vi "AudioTest.Load All Plot Limit Definition Files.vi"(8 "error in (no error)":errorcluster, 11 "Config Folder":path=path "C:/MTE/Audio Test/Config") -> (0 "error out":errorcluster, 3 "LimitPlots":T1[](array[typedef]))   [LabVIEW 2018]
uses:
  TypeDefs/AudioTest.Result Plot Data.ctl
  <vilib>/KATE/Files/File Utils.lvlib
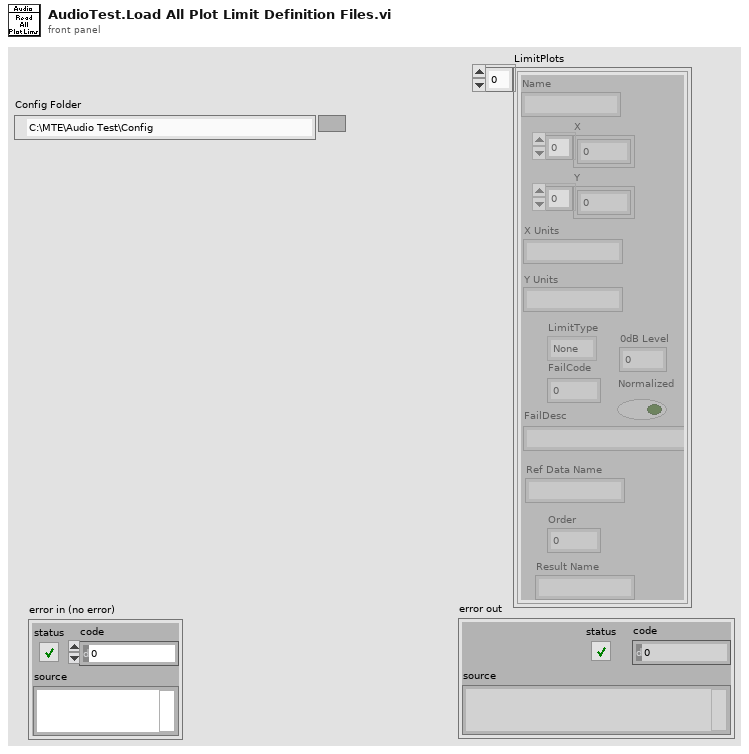
[diagram p1: front panel]
types:
  T1 = typedef "AudioTest.Result Plot Data.ctl" = cluster{"Order":i32, "Name":string, "X":dbl[], "Y":dbl[], "X Units":string, "Y Units":string, "LimitType":enum16{"None", "LL", "UL"}, "FailCode":i32, "FailDesc":string, "Ref Data Name":string, "Result Name":string, "0dB Level":dbl, "Normalized":bool}
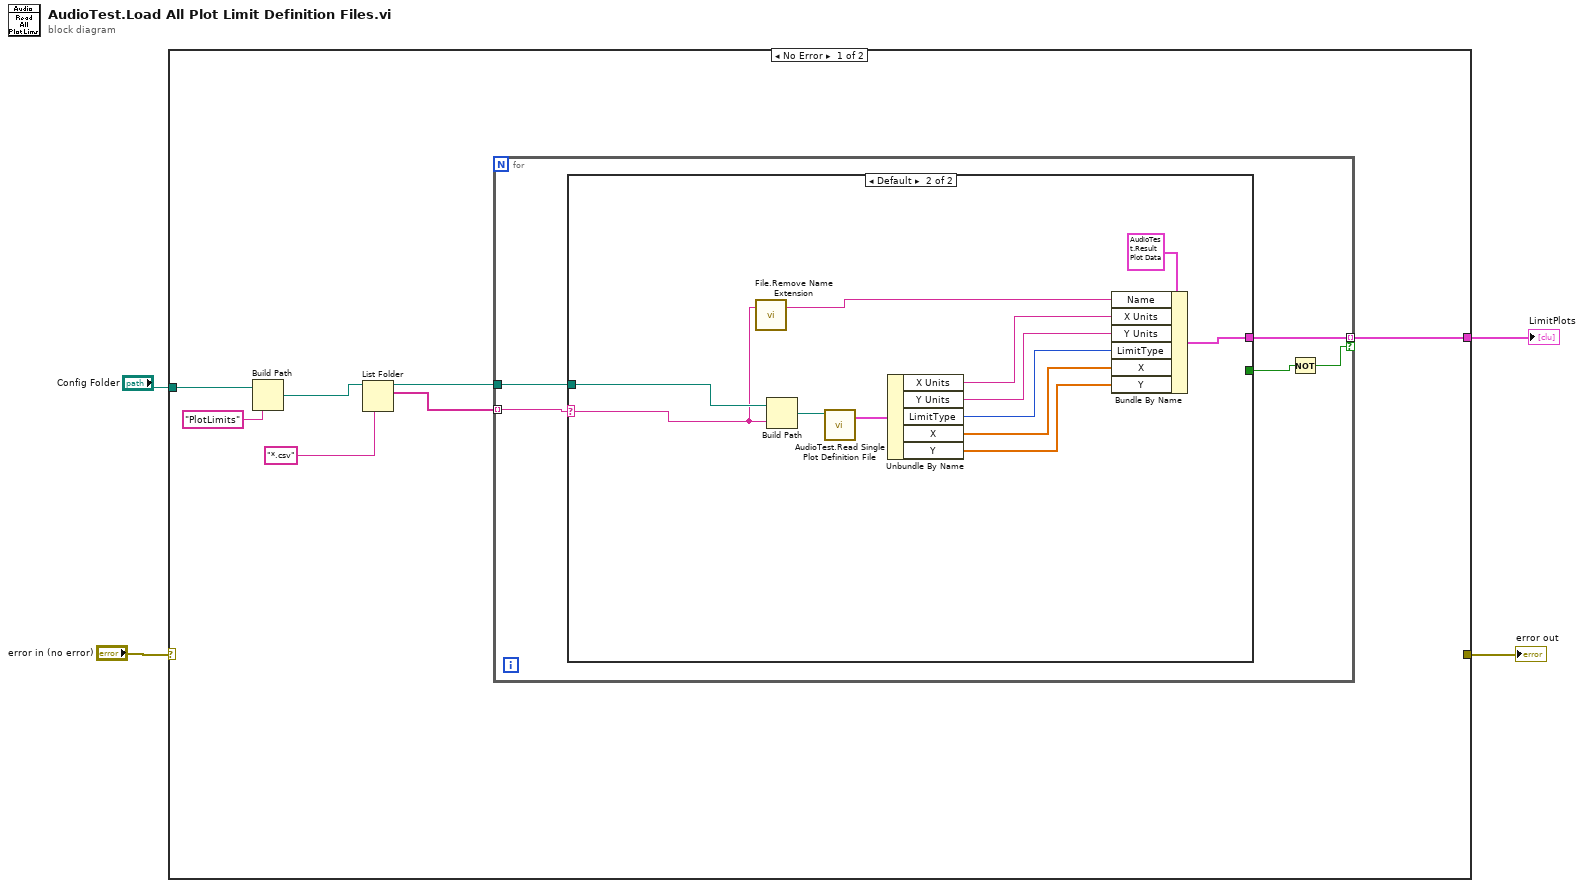
[diagram p0: block diagram]
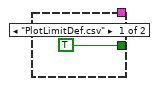
[diagram p2: hidden frame]
diagram:
  n1 = case shown="No Error" "error in (no error)" {
    selector: "error in (no error)" -> [_ w30]
    tunnel: "Config Folder" -> [w11 _]
    tunnel: [w9 _] -> w3
    tunnel: [_ w30] -> w1
    frame No Error {
      n2 = Build Path(base path=w11, name or relative path="PlotLimits") -> (appended path=w8:path)
      n3 = List Folder(path=w8, pattern="*.csv" ("name or relative path")) -> (path out=w6:path, filenames=w5:string[])  [unwired: 2 in, 2 out]
      n4 = for {
        tunnel: [w16] -> w9 mode=indexing if=w15
        tunnel: w6 -> [w13]
        tunnel: w5 -> [w12] mode=indexing
        n5 = case shown="Default" w12 {
          selector: w12 -> [_ w19]
          tunnel: [_ w22] -> w16
          tunnel: [TRUE _] -> w14
          tunnel: w13 -> [_ w20]
          frame "PlotLimitDef.csv" {
          }
          frame Default {
            n6 = call <vilib>:"File.Remove Name Extension.vi"("File Name"=w19) -> ("Name Less Ext"=w18:string)  [unwired: 1 in, 1 out]
            n7 = Build Path(base path=w20, name or relative path=w19) -> (appended path=w21:path)
            n8 = call "AudioTest.Read Single Plot Definition File.vi"("CSV File"=w21) -> ("Plot"=w28:T1)  [unwired: 9 in, 1 out]
            n9 = Unbundle By Name(w28) -> ("X Units"=w27:string, "Y Units"=w26:string, "LimitType"=w25:enum16{"None", "LL", "UL"}, "X"=w24:dbl[], "Y"=w23:dbl[])
            n10 = Bundle By Name(cluster=T1 {"Order"=0, "Name"="", "X"=[], "Y"=[], "X Units"="", "Y Units"="", "LimitType"=enum."None", "FailCode"=0, "FailDesc"="", "Ref Data Name"="", "Result Name"="", "0dB Level"=0.0, "Normalized"=FALSE}, "Name"=w18, "X Units"=w27, "Y Units"=w26, "LimitType"=w25, "X"=w24, "Y"=w23) -> (w22:T1)
          }
        }
        n11 = Not(x=w14) -> (.not. x?=w15:bool)
      }
    }
    frame Error {
    }
  }
  "LimitPlots" <- w3
  "error out" <- w1
